vi "solar_write ThisCtrls.vi"(8 "error in (no error)":errorcluster, 10 "Ctrls":refnum<vi>[](array[refnum]), 11 "solar in":refnum<class "solar.lvclass">) -> (0 "error out":errorcluster, 3 "solar out":refnum<class "solar.lvclass">)   [LabVIEW 2018, in "solar.lvclass"]
doc: "This sets the control references used to load/reload the last known values during initialization and shutdown."
uses:
  solar.lvclass
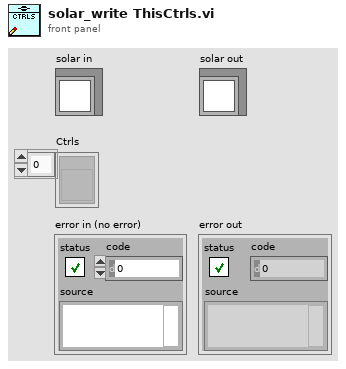
[diagram p1: front panel]
types:
  T1 = typedef "solar_ctl SOLAR Refnum.ctl" = refnum<k1>
  T2 = typedef "solar_ctl SOLAR Global.ctl" = cluster{"Targets":T3[], "AppDir":path, "solar.ini":path, "ConfigsDir":path, "CosmosDir":path, "LogsDir":path, "ExePath":path, "ExeVersion":string, "PartNum":string, "AppSetup":string, "Title":string, "Main.ini":path, "Temp.ini":path, "vSOLAR":string, "Splash.png":string, "SplashWait":i32, "SOLARUE":refnum<user-event>, "VoyagerRefnum":T4, "QTimerRefnum":T5}
  T3 = typedef "solar_ctl Target Global.ctl" = cluster{"Target":string, "Q":refnum<queue>, "UE":refnum<user-event>, "VI":refnum<vi>, "Menu":refnum<k9>, "Data":refnum<data-value>, "Attributes":variant}
  T4 = typedef "solar_voy_ctl Voyager Refnum.ctl" = refnum<k1>
  T5 = typedef "solar_qtimer_ctl Refnum.ctl" = refnum<k1>
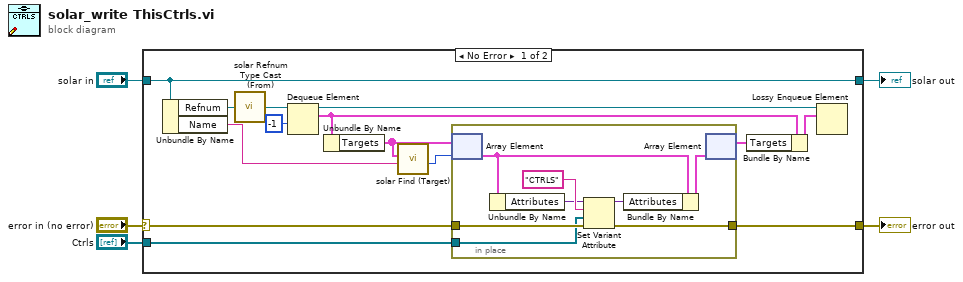
[diagram p0: block diagram]
diagram:
  n1 = case shown="No Error" "error in (no error)" {
    selector: "error in (no error)" -> [w18 w29]
    tunnel: "solar in" -> [w19 w28]
    tunnel: [w15 w29] -> w5
    tunnel: [w19 w28] -> w4
    tunnel: "Ctrls" -> [w6 _]
    frame No Error {
      n2 = Unbundle By Name(w19) -> ("Refnum"=w17:T1, "Name"=w14:string)
      n3 = call "solar Refnum Type Cast (From).vi"("Refnum"=w17) -> ("SOLAR"=w16:refnum<queue>)
      n4 = Dequeue Element(queue=w16, timeout in ms (-1)=-1) -> (queue out=w13:refnum<queue>, element=w11:T2)  [unwired: 1 in, 2 out]
      n5 = Unbundle By Name(w11) -> ("Targets"=w7:T3[])
      n6 = call "solar Find (Target).vi"("Target"=w14, "Targets"=w7) -> ("Target Index"=w9:i32)  [unwired: 8 in, 1 out]
      n7 = in-place {
        in-place-border: w18 -> [w21]
        in-place-border: [w24] -> w15
        in-place-border: w6 -> [w20]
        n8 = in-place-array #1(w7, w9) -> (w27:T3)
        n9 = Unbundle By Name(w27) -> ("Attributes"=w22:variant)
        n10 = Set Variant Attribute(Variant=w22, name="CTRLS", value=w20, error in=w21) -> (Variant out=w25:variant, error out=w24:errorcluster)  [unwired: 1 out]
        n11 = Bundle By Name(cluster=w27, "Attributes"=w25) -> (w26:T3)
        n12 = in-place-array #1(w26) -> (w8:T3[])  [unwired: 1 out]
      }
      n13 = Bundle By Name(cluster=w11, "Targets"=w8) -> (w10:T2)
      n14 = Lossy Enqueue Element(queue=w13, element=w10) -> ()  [unwired: 1 in, 4 out]
    }
    frame Error {
    }
  }
  "error out" <- w5
  "solar out" <- w4
